vi "ParameterString Replace.vi"(0 "String":string="PPC_Enabled=YES\nPPC_EXID[0]=0x09\nPPC_EXID[1]=0x00\nPPC_EXID[2]=0x02\nPOP1_Enabled=NO\nPOP1_EXID[0]=0x00\nPOP1_EXID[1]=0x00\nPOP1_EXID[2]=0x00\nPOP2_Enabled=NO\nPOP2_EXID[0]=0x00\nPOP2_EXID[1]=0x00\nPOP2_EXID[2]=0x00\nPPC_Text=Default PPC\nPulseWidthStep=100\nAmplitudeSteps=50\nPPC_AllowIndividualPulseAmplMod=YES\nPPC_AllowIndividualPulseWidthMod=YES\nPPC_AllowProgramFreqMod=YES\nIPG_MagnetOptions_Behavior_A_Enabled=YES\nIPG_MagnetOptions_Behavior_B_Enabled=NO\nIPG_MagnetOptions_Behavior_C_Enabled=NO\nImplantDateTime=MM/DD/YYYY 00:00:00 PM\nReplacementIntervalMonths=60", 1 "Key":string="PulseWidthStep", 2 "New Value":string="1234", 12 "TermChars":string="\r\n") -> (4 "Updated String":string="PPC_Enabled=YES\nPPC_EXID[0]=0x09\nPPC_EXID[1]=0x00\nPPC_EXID[2]=0x02\nPOP1_Enabled=NO\nPOP1_EXID[0]=0x00\nPOP1_EXID[1]=0x00\nPOP1_EXID[2]=0x00\nPOP2_Enabled=NO\nPOP2_EXID[0]=0x00\nPOP2_EXID[1]=0x00\nPOP2_EXID[2]=0x00\nPPC_Text=Default PPC\nPulseWidthStep=1234\nAmplitudeSteps=50\nPPC_AllowIndividualPulseAmplMod=YES\nPPC_AllowIndividualPulseWidthMod=YES\nPPC_AllowProgramFreqMod=YES\nIPG_MagnetOptions_Behavior_A_Enabled=YES\nIPG_MagnetOptions_Behavior_B_Enabled=NO\nIPG_MagnetOptions_Behavior_C_Enabled=NO\nImplantDateTime=MM/DD/YYYY 00:00:00 PM\nReplacementIntervalMonths=60", 8 "Old Value":string="100", 10 "Found":bool=TRUE)   [LabVIEW 2010]
doc: "This VI expects a (\\r\\n) line-terminated multipline String composed of Key = Value pairs, such as:\n\naKey1=value1(\\r\\n)\naKey2=value2(\\r\\n)\n.......\n\nNew Value is the replacement value for your Key.\nOld Value is the value that was initial found before being replaced.\nFound is true if Key was found in String."
panel:
  # "="
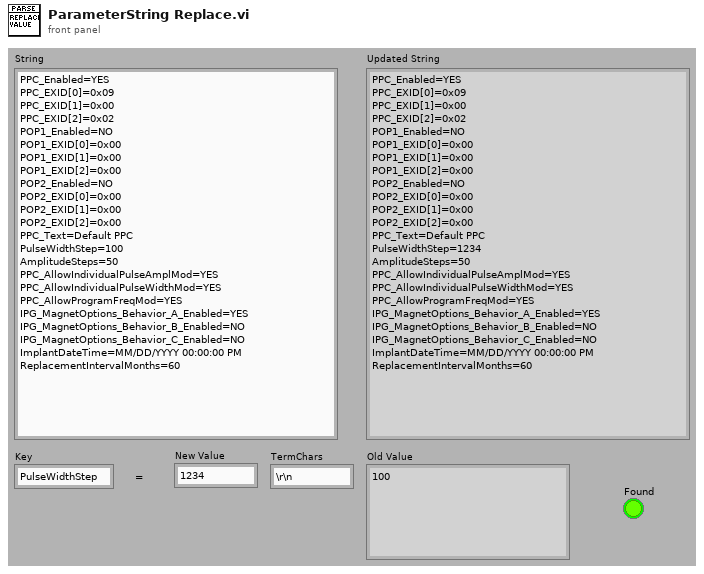
[diagram p1: front panel]
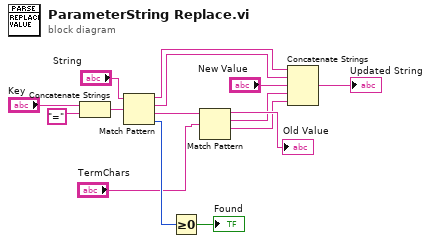
[diagram p0: block diagram]
diagram:
  n1 = Concatenate Strings("Key", "=" ("string")) -> (w12:string)
  n2 = Match Pattern(string="String", regular expression=w12) -> (before substring=w9:string, match substring=w8:string, after substring=w11:string, offset past match=w3:i32)  [unwired: 1 in]
  n3 = Greater Or Equal To 0?(x=w3) -> (x >= 0?=→"Found":bool)
  n4 = Match Pattern(string=w11, regular expression="TermChars") -> (before substring=→"Old Value":string, match substring=w6:string, after substring=w5:string)  [unwired: 1 in, 1 out]
  n5 = Concatenate Strings(w9, w8, "New Value", w6, w5) -> (→"Updated String":string)
